vi "Autonomous Independent.vi"() -> ()   [LabVIEW 2016]
doc: "This VI is called when autonomous begins, and will automatically be terminated when autonomous ends. You can carry out timed or sensor driven robot movement independently without needing to return to the caller."
uses:
  <vilib>/Rock Robotics/WPI/Solenoid/WPI_SolenoidValue.ctl
  <vilib>/Rock Robotics/Network Tables/NT Read String.vi
  <vilib>/Rock Robotics/WPI/Solenoid/WPI_SolenoidSetEnum.vi
panel:
  in  "Target Angle":dbl
  out "Refnum's Out":T1
  in  "Target Distance":dbl=15.0 format="%#_13g"
  out "Error Out":errorcluster
  in  "Error In":errorcluster
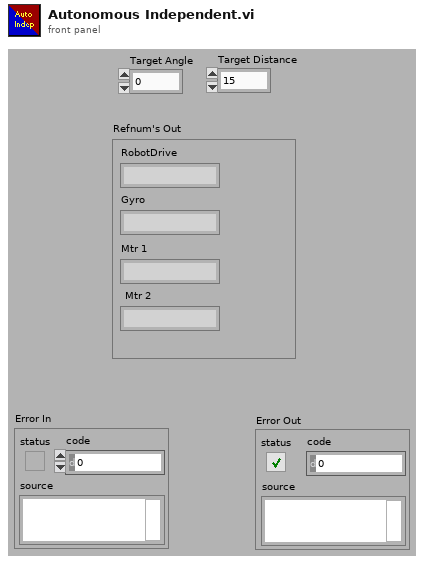
[diagram p1: front panel]
types:
  T1 = cluster{"RobotDrive":string, "Gyro":string, "Mtr 1":string, "Mtr 2":string}
  T2 = typedef "WPI_SolenoidValue.ctl" = enum16{"Off", "On", "Forward", "Reverse"}
  T3 = cluster{"Gyro":string, "Mtr 1":string, "Mtr 2":string}
  T4 = typedef "WPI_MotorControlDeviceRef.ctl" = cluster{"DeviceStatus":errorcluster, "Type":T5, "PWM":cluster{"PWM Channel":T6, "DeadBand":T7}, "CAN":cluster{"Device Number":u8, "SetOutput VI Ref":variant, "GetOutput VI Ref":variant, "Enable VI Ref":variant, "Disable VI Ref":variant, "Data":variant}, "Invert":bool}
  T5 = typedef "WPI_MotorControlType.ctl" = enum16{"PWM", "CAN"}
  T6 = typedef "FPGA_DIOPWMChannel.ctl" = enum8{"PWM 0", "PWM 1", "PWM 2", "PWM 3", "PWM 4", "PWM 5", "PWM 6", "PWM 7", "PWM 8", "PWM 9", "PWM MXP 0", "PWM MXP 1", "PWM MXP 2", "PWM MXP 3", "PWM MXP 4", "PWM MXP 5", "PWM MXP 6", "PWM MXP 7", "PWM MXP 8", "PWM MXP 9", "Invalid"}
  T7 = typedef "WPI_PWMDeadband.ctl" = cluster{"Name":string, "maxPositivePwm":i32, "minPositivePwm":i32, "centerPwm":i32, "maxNegativePwm":i32, "minNegativePwm":i32, "angularRange":u16}
  T8 = typedef "WPI_GyroDevRef.ctl" = cluster{"DevStatus":errorcluster, "Analog Channel":T9, "Offset":dbl, "Gain (VoltsPerDegree/Second)":dbl, "Gyro Type":enum16{"Analog", "XRS450"}, "Handle":i32, "SPI Bus":T10, "Device Found":bool, "Sample Rate":dbl, "Calibrate On Open":bool}
  T9 = typedef "FPGA_AIChannel.ctl" = enum8{"AI 0", "AI 1", "AI 2", "AI 3", "AI MXP 0", "AI MXP 1", "AI MXP 2", "AI MXP 3", "Invalid"}
  T10 = typedef "spi_bus.ctl" = enum16{"SPI On-Board, CS0", "SPI On-Board, CS1", "SPI On-Board, CS2", "SPI On-Board, CS3", "SPI MXP", "Invalid"}
  T11 = typedef "WPI_SolenoidDevRef.ctl" = cluster{"DevStatus":errorcluster, "Pneumatics Control Module":u8, "Forward Solenoid Channel":T12, "Reverse Solenoid Channel":T12}
  T12 = typedef "WPI_SolenoidChannel.ctl" = enum8{"Solenoid 0", "Solenoid 1", "Solenoid 2", "Solenoid 3", "Solenoid 4", "Solenoid 5", "Solenoid 6", "Solenoid 7", "Invalid"}
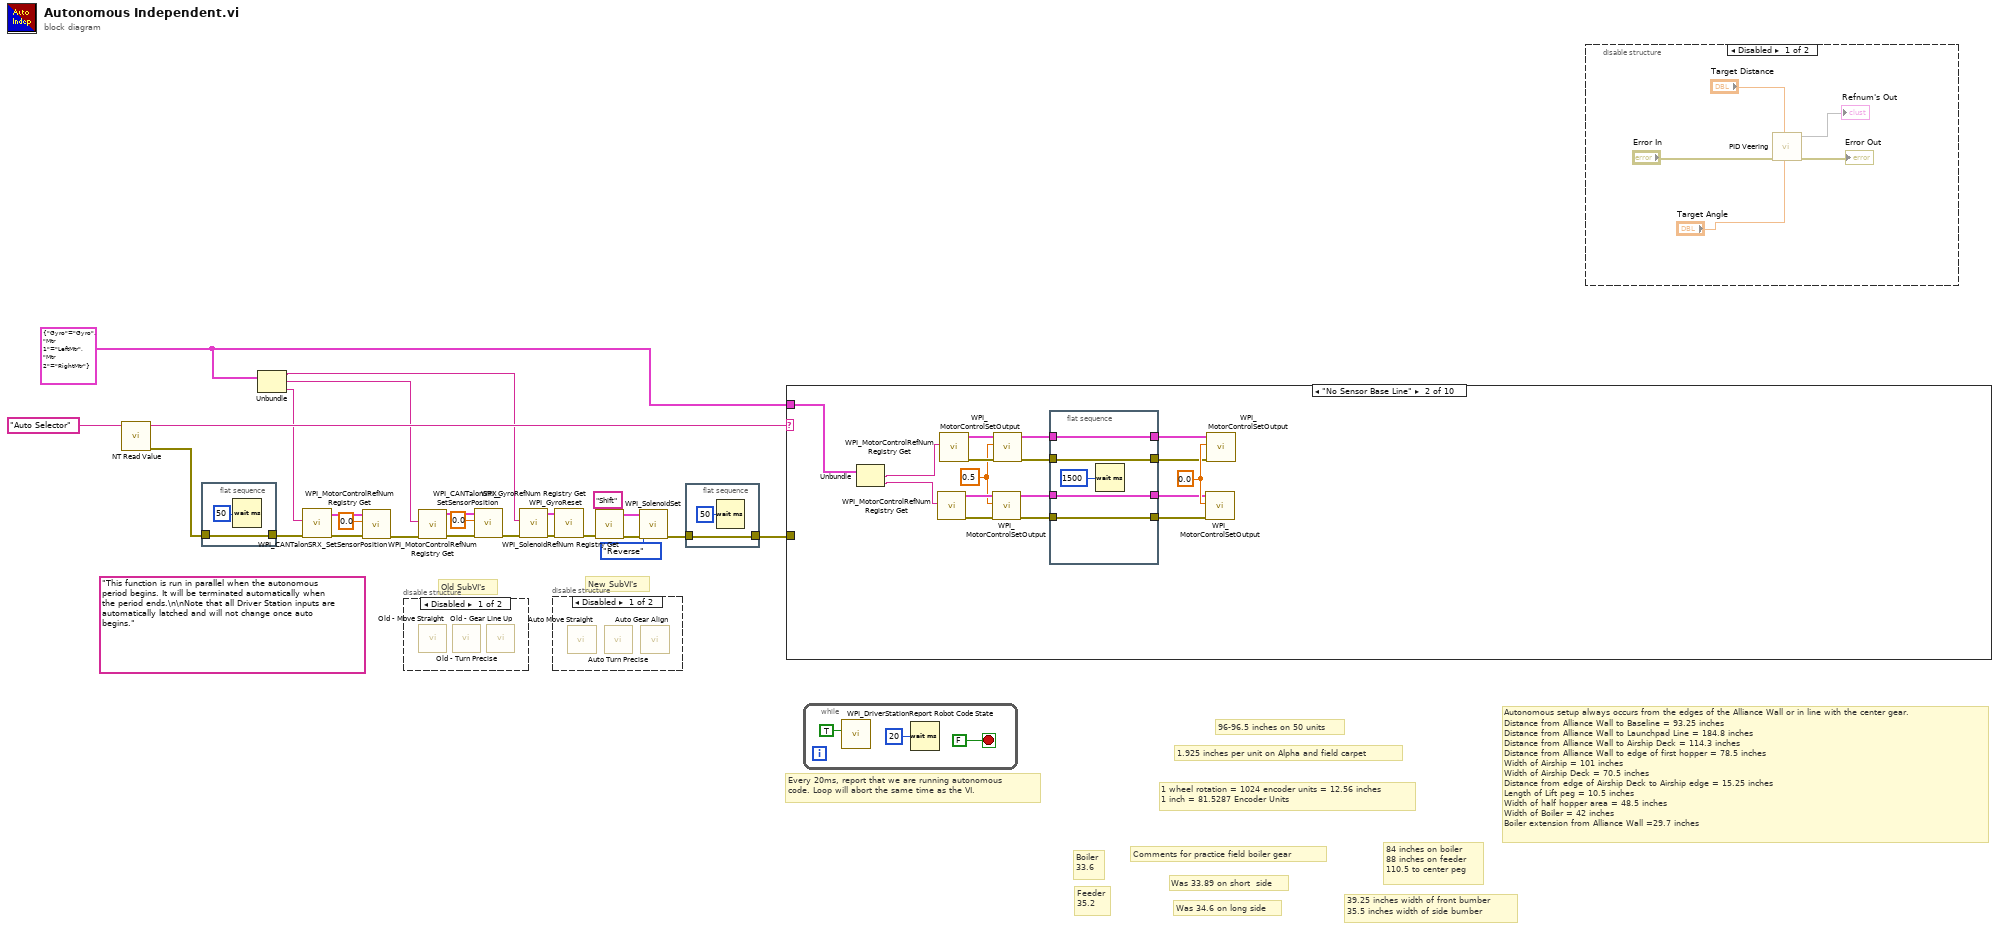
[diagram p0: block diagram]
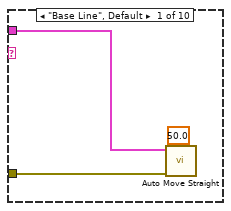
[diagram p3: hidden frame]
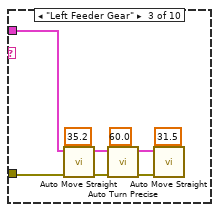
[diagram p4: hidden frame]
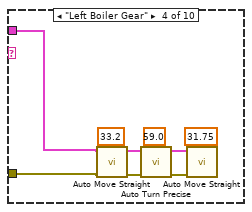
[diagram p5: hidden frame]
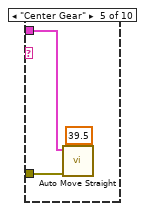
[diagram p6: hidden frame]
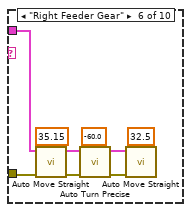
[diagram p7: hidden frame]
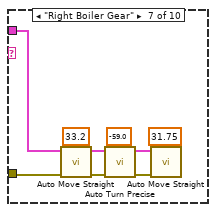
[diagram p8: hidden frame]
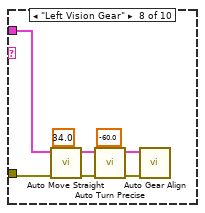
[diagram p9: hidden frame]
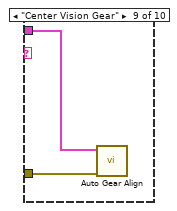
[diagram p10: hidden frame]
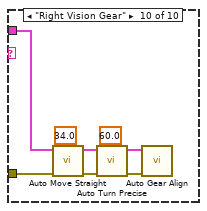
[diagram p11: hidden frame]
diagram:
  w5 = T3 {"Gyro"="Gyro", "Mtr 1"="LeftMtr", "Mtr 2"="RightMtr"} ("Refnum's")
  (unwired) "This function is run in parallel when the autonomous period begins. It will be terminated automatically when the period ends.\n\nNote that all Driver Station inputs are automatically latched and will not change once auto begins."
  # "39.25 inches width of front bumber\n35.5 inches width of side bumber"
  # "84 inches on boiler\n88 inches on feeder \n110.5 to center peg"
  # "1.925 inches per unit on Alpha and field carpet"
  # "96-96.5 inches on 50 units"
  # "Feeder\n35.2"
  # "Boiler\n33.6"
  # "Comments for practice field boiler gear"
  # "Was 34.6 on long side"
  # "Was 33.89 on short  side"
  # "New SubVI's"
  # "Old SubVI's"
  # "Autonomous setup always occurs from the edges of the Alliance Wall or in line with the center gear.\nDistance from Alliance Wall to Baseline = 93.25 inches\nDistance from Alliance Wall to Launchpad Line = 184.8 inches\nDistance from Alliance Wall to Airship Deck = 114.3 inches\nDistance from Alliance Wall to edge of first hopper = 78.5 inches\nWidth of Airship = 101 inches\nWidth of Airship Deck = 70.5 inches\nDistance from edge of Airship Deck to Airship edge = 15.25 inches\nLength of Lift peg = 10.5 inches\nWidth of half hopper area = 48.5 inches\nWidth of Boiler = 42 inches\nBoiler extension from Alliance Wall =29.7 inches"
  # "1 wheel rotation = 1024 encoder units = 12.56 inches\n1 inch = 81.5287 Encoder Units"
  # "Every 20ms, report that we are running autonomous\ncode. Loop will abort the same time as the VI."
  n1 = call-poly <vilib>:"NT Read Value.vi"("Name"="Auto Selector") -> ("error out"=w23:errorcluster, "String"=w24:string)  [unwired: 9 in]
  n2 = flat-sequence {
    tunnel: [w26] -> w9
    tunnel: w23 -> [w26]
    frame #0 {
      n3 = Wait (ms)(milliseconds to wait=u32 50) -> ()  [unwired: 1 out]
    }
  }
  n4 = Unbundle(w5) -> ("Gyro"=w4:string, "Mtr 1"=w3:string, "Mtr 2"=w2:string)
  n5 = call <vilib>:"WPI_MotorControlRefNum Registry Get.vi"("error in (no error)"=w9, "refnum name"=w2) -> ("error out"=w11:errorcluster, "MotorControlDevRef"=w12:T4)  [unwired: 8 in]
  n6 = call <vilib>:"WPI_CANTalonSRX_SetSensorPosition.vi"("error in (no error)"=w11, "New Sensor Position"=0.0, "CAN Talon SRX Ref"=w12) -> ("error out"=w8:errorcluster)  [unwired: 7 in, 1 out]
  n7 = disable-structure shown="Disabled" {
    frame Disabled {
      n8 = call "Old - Move Straight.vi"() -> ()  [unwired: 11 in, 1 out]
      n9 = call "Old - Turn Precise.vi"() -> ()  [unwired: 11 in, 1 out]
      n10 = call "Old - Gear Line Up.vi"() -> ()  [unwired: 11 in, 1 out]
    }
    frame Enabled {
    }
  }
  n11 = call <vilib>:"WPI_MotorControlRefNum Registry Get.vi"("error in (no error)"=w8, "refnum name"=w3) -> ("error out"=w14:errorcluster, "MotorControlDevRef"=w15:T4)  [unwired: 8 in]
  n12 = call <vilib>:"WPI_CANTalonSRX_SetSensorPosition.vi"("error in (no error)"=w14, "New Sensor Position"=0.0, "CAN Talon SRX Ref"=w15) -> ("error out"=w7:errorcluster)  [unwired: 7 in, 1 out]
  n13 = call <vilib>:"WPI_GyroRefNum Registry Get.vi"("error in (no error)"=w7, "refnum name"=w4) -> ("error out"=w22:errorcluster, "GyroDevRef"=w21:T8)  [unwired: 8 in]
  n14 = disable-structure shown="Disabled" {
    frame Disabled {
      n15 = call "Auto Move Straight.vi"() -> ()  [unwired: 10 in, 2 out]
      n16 = call "Auto Turn Precise.vi"() -> ()  [unwired: 10 in, 2 out]
      n17 = call "Auto Gear Align.vi"() -> ()  [unwired: 10 in, 2 out]
    }
    frame Enabled {
    }
  }
  n18 = call <vilib>:"WPI_GyroReset.vi"("error in"=w22, "GyroDevRef"=w21) -> ("error out"=w16:errorcluster)  [unwired: 8 in, 1 out]
  n19 = call <vilib>:"WPI_SolenoidRefNum Registry Get.vi"("error in (no error)"=w16, "refnum name"="Shift") -> ("error out"=w20:errorcluster, "SolenoidDevRef"=w19:T11)  [unwired: 8 in]
  n20 = call-poly <vilib>:"WPI_SolenoidSet.vi"("error in (no error)"=w20, "Value"=WPI_SolenoidValue."Reverse", "SolenoidDevRef"=w19) -> ("error out"=w6:errorcluster)  [unwired: 7 in, 1 out]
  n21 = flat-sequence {
    tunnel: [w28] -> w1
    tunnel: w6 -> [w28]
    frame #0 {
      n22 = Wait (ms)(milliseconds to wait=u32 50) -> ()  [unwired: 1 out]
    }
  }
  n23 = case shown="\"No Sensor Base Line\"" w24 {
    tunnel: w5 -> [w32 w35 w58 w66 w74 w76 w86 w94 w102 w104]
    tunnel: w1 -> [w31 _ w59 w67 w75 w77 w87 w95 w103 w105]
    frame "Base Line", Default {
      n24 = call "Auto Move Straight.vi"("Target Distance"=50.0, "Error In"=w31, "Refnum's In"=w32) -> ()  [unwired: 7 in, 2 out]
    }
    frame "No Sensor Base Line" {
      w44 = 0.0 ("Output")
      w45 = 0.5 ("Output")
      n25 = Unbundle(w35) -> ("Mtr 1"=w34:string, "Mtr 2"=w33:string)  [unwired: 1 out]
      n26 = call <vilib>:"WPI_MotorControlRefNum Registry Get.vi"("refnum name"=w33) -> ("error out"=w48:errorcluster, "MotorControlDevRef"=w49:T4)  [unwired: 9 in]
      n27 = call <vilib>:"WPI_MotorControlRefNum Registry Get.vi"("refnum name"=w34) -> ("error out"=w47:errorcluster, "MotorControlDevRef"=w46:T4)  [unwired: 9 in]
      n28 = call <vilib>:"WPI_MotorControlSetOutput.vi"("error in (no error)"=w48, "Output"=w45, "MotorControlDevRef"=w49) -> ("error out"=w38:errorcluster, "MotorControlDevRef"=w42:T4)  [unwired: 6 in, 1 out]
      n29 = call <vilib>:"WPI_MotorControlSetOutput.vi"("error in (no error)"=w47, "Output"=w45, "MotorControlDevRef"=w46) -> ("error out"=w37:errorcluster, "MotorControlDevRef"=w41:T4)  [unwired: 6 in, 1 out]
      n30 = flat-sequence {
        tunnel: [w53] -> w43
        tunnel: w42 -> [w53]
        tunnel: w41 -> [w52]
        tunnel: [w52] -> w40
        tunnel: [w51] -> w39
        tunnel: w38 -> [w51]
        tunnel: w37 -> [w50]
        tunnel: [w50] -> w36
        frame #0 {
          n31 = Wait (ms)(milliseconds to wait=u32 1500) -> ()  [unwired: 1 out]
        }
      }
      n32 = call <vilib>:"WPI_MotorControlSetOutput.vi"("error in (no error)"=w39, "Output"=w44, "MotorControlDevRef"=w43) -> ()  [unwired: 6 in, 3 out]
      n33 = call <vilib>:"WPI_MotorControlSetOutput.vi"("error in (no error)"=w36, "Output"=w44, "MotorControlDevRef"=w40) -> ()  [unwired: 6 in, 3 out]
    }
    frame "Left Feeder Gear" {
      n34 = call "Auto Move Straight.vi"("Target Distance"=35.2, "Error In"=w59, "Refnum's In"=w58) -> ("Error Out"=w63:errorcluster, "Refnum's Out"=w62:T3)  [unwired: 7 in]
      n35 = call "Auto Turn Precise.vi"("Target Distance"=60.0, "Error In"=w63, "Refnum's In"=w62) -> ("Error Out"=w61:errorcluster, "Refnum's Out"=w60:T3)  [unwired: 7 in]
      n36 = call "Auto Move Straight.vi"("Target Distance"=31.5, "Error In"=w61, "Refnum's In"=w60) -> ()  [unwired: 7 in, 2 out]
    }
    frame "Left Boiler Gear" {
      n37 = call "Auto Move Straight.vi"("Target Distance"=33.2, "Error In"=w67, "Refnum's In"=w66) -> ("Error Out"=w72:errorcluster, "Refnum's Out"=w71:T3)  [unwired: 7 in]
      n38 = call "Auto Turn Precise.vi"("Target Distance"=59.0, "Error In"=w72, "Refnum's In"=w71) -> ("Error Out"=w70:errorcluster, "Refnum's Out"=w69:T3)  [unwired: 7 in]
      n39 = call "Auto Move Straight.vi"("Target Distance"=31.75, "Error In"=w70, "Refnum's In"=w69) -> ()  [unwired: 7 in, 2 out]
    }
    frame "Center Gear" {
      n40 = call "Auto Move Straight.vi"("Target Distance"=39.5, "Error In"=w75, "Refnum's In"=w74) -> ()  [unwired: 7 in, 2 out]
    }
    frame "Right Feeder Gear" {
      n41 = call "Auto Move Straight.vi"("Target Distance"=35.15, "Error In"=w77, "Refnum's In"=w76) -> ("Error Out"=w78:errorcluster, "Refnum's Out"=w79:T3)  [unwired: 7 in]
      n42 = call "Auto Turn Precise.vi"("Target Distance"=-60.0, "Error In"=w78, "Refnum's In"=w79) -> ("Error Out"=w80:errorcluster, "Refnum's Out"=w81:T3)  [unwired: 7 in]
      n43 = call "Auto Move Straight.vi"("Target Distance"=32.5, "Error In"=w80, "Refnum's In"=w81) -> ()  [unwired: 7 in, 2 out]
    }
    frame "Right Boiler Gear" {
      n44 = call "Auto Move Straight.vi"("Target Distance"=33.2, "Error In"=w87, "Refnum's In"=w86) -> ("Error Out"=w88:errorcluster, "Refnum's Out"=w89:T3)  [unwired: 7 in]
      n45 = call "Auto Turn Precise.vi"("Target Distance"=-59.0, "Error In"=w88, "Refnum's In"=w89) -> ("Error Out"=w90:errorcluster, "Refnum's Out"=w91:T3)  [unwired: 7 in]
      n46 = call "Auto Move Straight.vi"("Target Distance"=31.75, "Error In"=w90, "Refnum's In"=w91) -> ()  [unwired: 7 in, 2 out]
    }
    frame "Left Vision Gear" {
      n47 = call "Auto Move Straight.vi"("Target Distance"=34.0, "Error In"=w95, "Refnum's In"=w94) -> ("Error Out"=w101:errorcluster, "Refnum's Out"=w100:T3)  [unwired: 7 in]
      n48 = call "Auto Turn Precise.vi"("Target Distance"=-60.0, "Error In"=w101, "Refnum's In"=w100) -> ("Error Out"=w97:errorcluster, "Refnum's Out"=w96:T3)  [unwired: 7 in]
      n49 = call "Auto Gear Align.vi"("Error In"=w97, "Refnum's In"=w96) -> ()  [unwired: 8 in, 2 out]
    }
    frame "Center Vision Gear" {
      n50 = call "Auto Gear Align.vi"("Error In"=w103, "Refnum's In"=w102) -> ()  [unwired: 8 in, 2 out]
    }
    frame "Right Vision Gear" {
      n51 = call "Auto Move Straight.vi"("Target Distance"=34.0, "Error In"=w105, "Refnum's In"=w104) -> ("Error Out"=w106:errorcluster, "Refnum's Out"=w107:T3)  [unwired: 7 in]
      n52 = call "Auto Turn Precise.vi"("Target Distance"=60.0, "Error In"=w106, "Refnum's In"=w107) -> ("Error Out"=w110:errorcluster, "Refnum's Out"=w111:T3)  [unwired: 7 in]
      n53 = call "Auto Gear Align.vi"("Error In"=w110, "Refnum's In"=w111) -> ()  [unwired: 8 in, 2 out]
    }
  }
  n54 = while {
    stop <- FALSE stop-if-true
    n55 = call <vilib>:"WPI_DriverStationReport Robot Code State.vi"("Autonomous"=TRUE) -> ()  [unwired: 10 in, 1 out]
    n56 = Wait (ms)(milliseconds to wait=u32 20) -> ()  [unwired: 1 out]
  }
  n57 = disable-structure shown="Disabled" {
    frame Disabled {
      n58 = call "PID Veering.vi"("Error"="Target Angle", "Current Distance"="Target Distance", "error in (no error)"="Error In") -> ("error out"=→"Error Out":errorcluster, 3:→"Refnum's Out")  [unwired: 7 in]
    }
    frame Enabled {
    }
  }
